vi "MODBUS_read_register_standalone.vi"(7 "MODBUS Serial Parameters":T1={"Mode"=enum."RTU", "Default Slave Address"=111, "MODBUS timeout"=1000, "Baud Rate"=38400, "Parity"=0, "Flow Control"=0} {"Parity" items=["None", "Odd", "Even", "Mark", "Space"]; "Flow Control" items=["None", "XON/XOFF", "RTS/CTS", "XON/XOFF & RTS/CTS", "DTR/DSR", "XON/XOFF & DTR/DSR"]}, 8 "error in":errorcluster, 9 "Register":u16=285, 10 "data type":u16(ring)=2 items=["U16", "U32", "F32", "A8", "A12", "A16", "A22"], 11 "VISA resource name":refnum<visa-resource-name>="MODBUS_485") -> (0 "error out":errorcluster, 1 "found?":bool, 2 "output cluster":cluster{"Numeric":u16, u32, "type single":sgl}, 3 "VISA resource name out":refnum<visa-resource-name>)   [LabVIEW 2012]
uses:
  NI Modbus.llb/MB Serial Master Query Read Holding Registers (poly).vi
  Manthey ModBus.llb/03 Read output registers.vi
panel:
  out "float out":sgl=496.2269
  out "U32 out":u32
  out "U16 out":u16
  out "Error Message":string
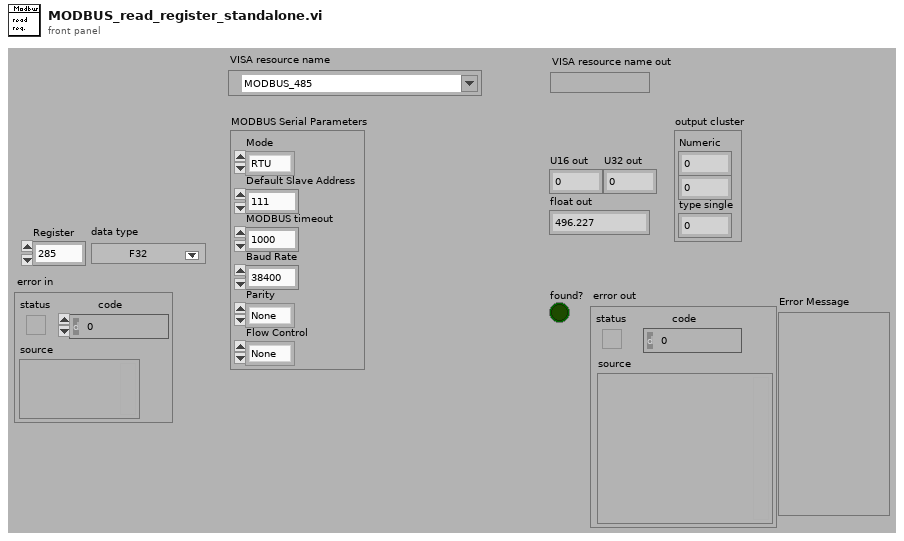
[diagram p1: front panel]
types:
  T1 = cluster{"Mode":enum16{"RTU", "ASCII"}, "Default Slave Address":u8, "MODBUS timeout":u32, "Baud Rate":u32, "Parity":u16, "Flow Control":u16}
  T2 = cluster{"Mode":enum16{"RTU", "ASCII"}, "Default Slave Address":u8}
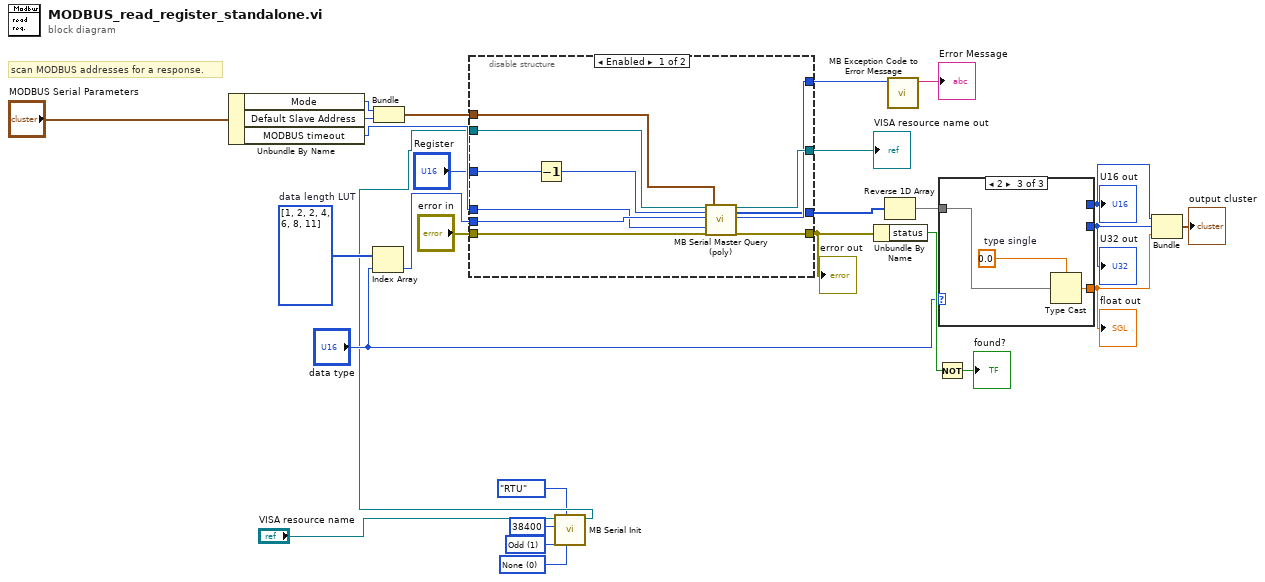
[diagram p0: block diagram]
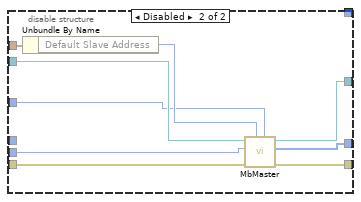
[diagram p2: hidden frame]
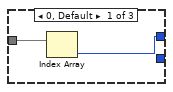
[diagram p3: hidden frame]
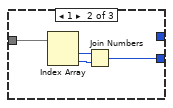
[diagram p4: hidden frame]
diagram:
  w2 = u16 0 items=["None", "XON/XOFF", "RTS/CTS", "XON/XOFF & RTS/CTS", "DTR/DSR", "XON/XOFF & DTR/DSR"] ("Flow Control")
  w3 = u16 1 items=["None", "Odd", "Even", "Mark", "Space"] ("Parity")
  w22 = u16[] [1, 2, 2, 4, 6, 8, 11]  # data length LUT
  # "scan MODBUS addresses for a response."
  n1 = Unbundle By Name("MODBUS Serial Parameters") -> ("Mode"=w12:enum16{"RTU", "ASCII"}, "Default Slave Address"=w11:u8, "MODBUS timeout"=w9:u32)
  n2 = Index Array(array=w22, index="data type") -> (element=w21:u16)
  n3 = Bundle("Mode"=w12, "Default Slave Address"=w11) -> (w10:T2)  [unwired: 1 in]
  n4 = call "MB Serial Init.vi"("Flow Control"=w2, "Mode"=enum16{"RTU", "ASCII"}."RTU", "Parity"=w3, "Baud Rate"=u32 38400, "VISA resource name"="VISA resource name") -> ("VISA resource name out"=w6:refnum<visa-resource-name>)  [unwired: 2 in, 4 out]
  n5 = disable-structure shown="Enabled" {
    disable-tunnel: [w39 w43] -> w27
    disable-tunnel: [w38 w45] -> w26
    disable-tunnel: [w37 _] -> w23
    disable-tunnel: "Register" -> [w30 w41]
    disable-tunnel: w21 -> [w36 w40]
    disable-tunnel: [w35 w44] -> w19
    disable-tunnel: w6 -> [w34 w46]
    disable-tunnel: "error in" -> [w33 w42]
    disable-tunnel: w10 -> [w32 w48]
    disable-tunnel: w9 -> [w31 _]
    frame Enabled {
      n6 = Decrement(x=w30) -> (x-1=w29:u16)
      n7 = call-poly "MB Serial Master Query (poly).vi"("VISA resource name"=w34, "Starting Address"=w29, "Quantity"=w36, "Timeout"=w31, "error in"=w33, "Serial Parameters"=w32) -> ("VISA resource name out"=w38:refnum<visa-resource-name>, "Holding Registers"=w35:u16[], "Exception Code"=w37:u8, "error out"=w39:errorcluster)  [unwired: 10 out]
    }
    frame Disabled {
      n8 = Unbundle By Name(w48) -> ("Default Slave Address"=w47:u8)
      n9 = call-poly "MbMaster.vi"("Protocol Start Address"=w41, "Modbus Slave Address"=w47, "error in (no error)"=w42, "Number of Points"=w40, "VISA resource name"=w46) -> ("error out"=w43:errorcluster, "Array of Registers"=w44:u16[], "VISA resource name out"=w45:refnum<visa-resource-name>)  [unwired: 3 in, 1 out]
    }
  }
  "error out" <- w27
  "VISA resource name out" <- w26
  n10 = Unbundle By Name(w27) -> ("status"=w25:bool)
  n11 = Reverse 1D Array(array=w19) -> (reversed array=w18:u16[])
  n12 = call "MB Exception Code to Error Message.vi"("Exception Code"=w23) -> ("Error Message"=→"Error Message":string)  [unwired: 10 in]
  n13 = Not(x=w25) -> (.not. x?=→"found?":bool)
  n14 = case shown="2" "data type" {
    tunnel: w18 -> [w50 w54 w56]
    tunnel: [w49 _ _] -> w16
    tunnel: [_ w51 _] -> w15
    tunnel: [_ _ w55] -> w14
    frame 0, Default {
      n15 = Index Array(array=w50) -> (element=w49:u16)  [unwired: 1 in]
    }
    frame 1 {
      n16 = Index Array(array=w54) -> (element #1=w53:u16, element #2=w52:u16)  [unwired: 2 in]
      n17 = Join Numbers(hi=w53, lo=w52) -> ((hi.lo)=w51:u32)
    }
    frame 2 {
      w57 = sgl 0.0  # type single
      n18 = Type Cast(type=w57, x=w56) -> (*(type *) &x=w55:sgl)
    }
  }
  "U16 out" <- w16
  "U32 out" <- w15
  "float out" <- w14
  n19 = Bundle("Numeric"=w16, w15, "type single"=w14) -> (→"output cluster":cluster{"Numeric":u16, u32, "type single":sgl})  [unwired: 1 in]
